vi "HaltRole.vi"(8 "error in (no error)":errorcluster, 10 "Game in":refnum<class "Game.lvclass">, 11 "HaltRole in":refnum<class "HaltRole.lvclass">) -> (0 "error out":errorcluster, 1 "Game out":refnum<class "Game.lvclass">, 2 "Robot out":refnum<class "Robot.lvclass">, 3 "HaltRole out":refnum<class "HaltRole.lvclass">)   [LabVIEW 2018, in "HaltRole.lvclass"]
uses:
  HaltRole.lvclass
  C:/Users/yugon/Desktop/SSL_AI/SSL_AI/Role_class/Role.lvclass
  Game_class/Game.lvclass
  Robot_class/Robot.lvclass
  Role_class/Role.lvclass/Role.ctl
  Tacticbook_class/Tacticbook.lvclass/Tacticbook.ctl
  HaltTactic_class/HaltTactic.lvclass/HaltTactic.ctl
  Tacticbook_class/Read HaltTactic.vi
  HaltTactic_class/Read States.vi
  Tacticbook_class/Write HaltTactic.vi
  Role_class/Read Tacticbook.vi
  Role_class/Write Tacticbook.vi
  Role_class/Write tactic_index.vi
  Role_class/Read RobotRef.vi
  Tacticbook_class/Tacticbook.lvclass
  HaltTactic_class/HaltTactic.lvclass
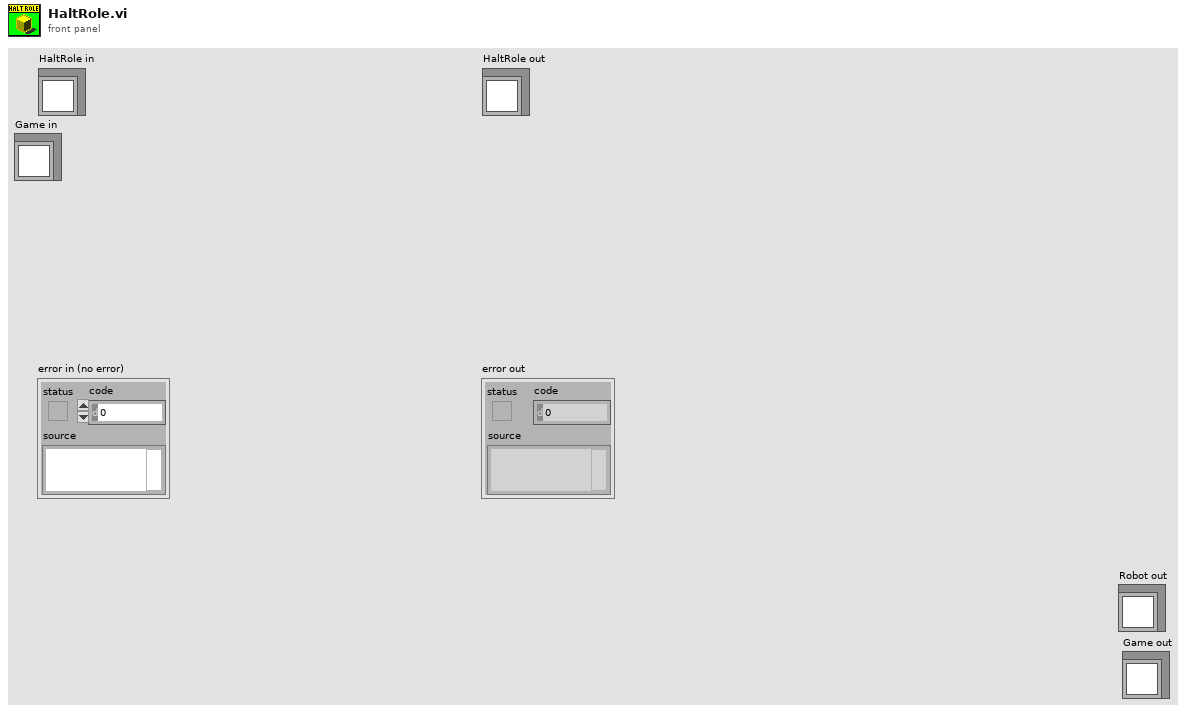
[diagram p1: front panel]
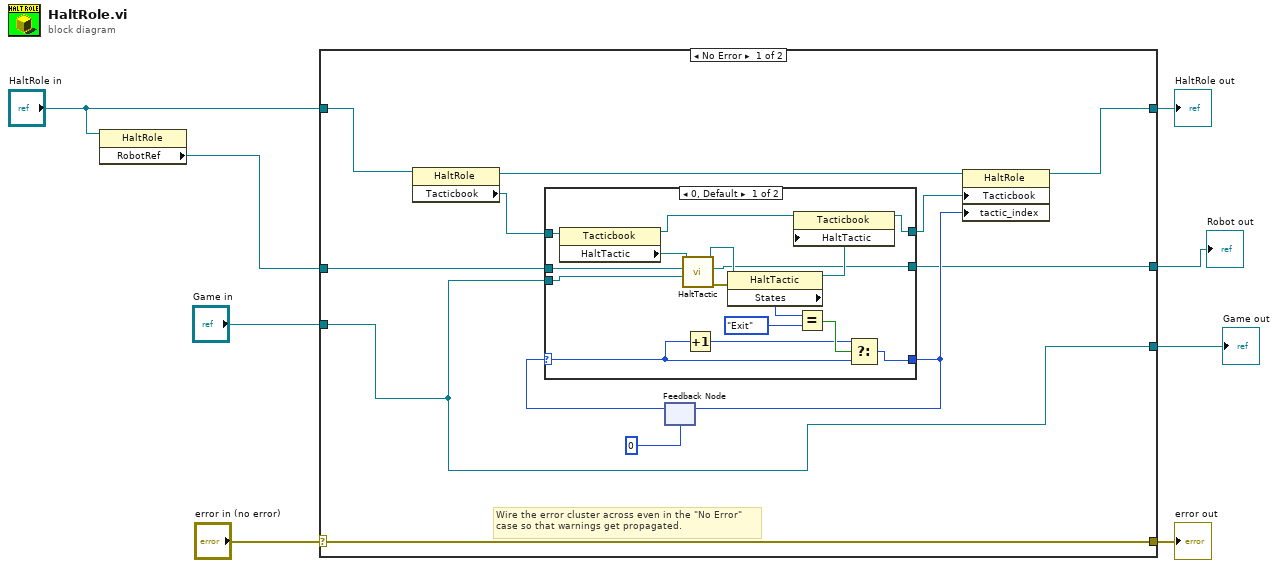
[diagram p0: block diagram]
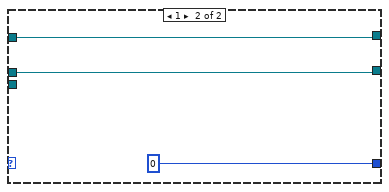
[diagram p2: hidden frame]
diagram:
  n1 = property class="HaltRole"(reference="HaltRole in") -> ("RobotRef"=w4:refnum<class "Robot.lvclass">)  [unwired: 1 in, 2 out]
  n2 = case shown="No Error" "error in (no error)" {
    selector: "error in (no error)" -> [w20 w43]
    tunnel: [w20 w43] -> w7
    tunnel: [w10 w42] -> w6
    tunnel: "HaltRole in" -> [w13 w42]
    tunnel: w4 -> [w12 w41]
    tunnel: "Game in" -> [w11 w40]
    tunnel: [w11 w40] -> w2
    tunnel: [w9 w41] -> w1
    frame No Error {
      # "Wire the error cluster across even in the \"No Error\"\ncase so that warnings get propagated."
      n3 = property class="HaltRole"(reference=w13) -> (reference out=w19:refnum<class "HaltRole.lvclass">, "Tacticbook"=w16:refnum<class "Tacticbook.lvclass">)  [unwired: 1 in, 1 out]
      n4 = feedback #1(0) -> (w17:i32)
      n5 = case shown="0, Default" w17 {
        selector: w17 -> [w29 _]
        tunnel: [w30 0] -> w15
        tunnel: w16 -> [w36 w38]
        tunnel: w11 -> [w23 _]
        tunnel: [w25 w38] -> w14
        tunnel: w12 -> [w24 w37]
        tunnel: [w22 w37] -> w9
        frame 0, Default {
          n6 = property class="Tacticbook"(reference=w36) -> (reference out=w27:refnum<class "Tacticbook.lvclass">, "HaltTactic"=w35:refnum<class "HaltTactic.lvclass">)  [unwired: 1 in, 1 out]
          n7 = call-dynamic "HaltTactic.vi"("Game in"=w23, "Robot"=w24, "HaltTactic in"=w35) -> ("error out"=w34:errorcluster, "Robot out"=w22:refnum<class "Robot.lvclass">, "HaltTactic out"=w33:refnum<class "HaltTactic.lvclass">)  [unwired: 6 in]
          n8 = Increment(x=w29) -> (x+1=w28:i32)
          n9 = property class="HaltTactic"(reference=w33, error in=w34) -> (reference out=w26:refnum<class "HaltTactic.lvclass">, "States"=w32:enum16{"Halt", "Exit"})  [unwired: 1 out]
          n10 = property class="Tacticbook"(reference=w27, "HaltTactic"=w26) -> (reference out=w25:refnum<class "Tacticbook.lvclass">)  [unwired: 1 in, 1 out]
          n11 = Equal?(x=w32, y=enum16{"Halt", "Exit"}."Exit") -> (x = y?=w31:bool)
          n12 = Select(t=w28, s=w31, f=w29) -> (s? t:f=w30:i32)
        }
        frame 1 {
        }
      }
      n13 = feedback-in #1(w15) -> ()
      n14 = property class="HaltRole"(reference=w19, "Tacticbook"=w14, "tactic_index"=w15) -> (reference out=w10:refnum<class "HaltRole.lvclass">)  [unwired: 1 in, 1 out]
    }
    frame Error {
    }
  }
  "error out" <- w7
  "HaltRole out" <- w6
  "Robot out" <- w1
  "Game out" <- w2
